vi "Start Tasks.vi"(8 "error in (no error)":errorcluster, 11 "Series Actor in":refnum<class "Series Actor.lvclass">) -> (0 "error out":errorcluster, 3 "Series Actor out":refnum<class "Series Actor.lvclass">)   [LabVIEW 2023, in "Series Actor.lvlib" / "Series Actor.lvclass"]
uses:
  Series Actor.lvclass
  C:/Program Files/National Instruments/LabVIEW 2023/vi.lib/ActorFramework/Actor/Actor.lvclass
  Task/Task Actor/Task Actor/Task Actor/Task Actor.lvclass
  Series Actor.lvclass/Series Actor.ctl
  Series Base/Series Base.lvclass/Series Base.ctl
  Task/Task Actor/Task Actor/Task Actor/Task Actor.lvclass/Task Actor.ctl
  <vilib>/ActorFramework/Message Enqueuer/Message Enqueuer.lvclass/Message Enqueuer.ctl
  <vilib>/ActorFramework/Message Enqueuer/Enqueue.vi
  Task/Task Actor/ITask Actor/ITask Actor Messages/Perform Action Msg/Perform Action Msg.lvclass
  C:/Program Files/National Instruments/LabVIEW 2023/vi.lib/ActorFramework/Message/Message.lvclass
  <vilib>/Utility/LVClass/Get LV Class Name.vi
  <resource>/AFDebug/Generate Trace for Message.vi
  <vilib>/ActorFramework/Message Priority Queue/Priority Enqueue.vi
  Series Base/Series Base.lvclass
  <vilib>/ActorFramework/Actor/Actor.lvclass
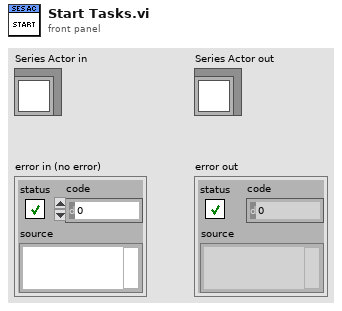
[diagram p1: front panel]
types:
  T1 = map{string, refnum<class "Message Enqueuer.lvclass">}
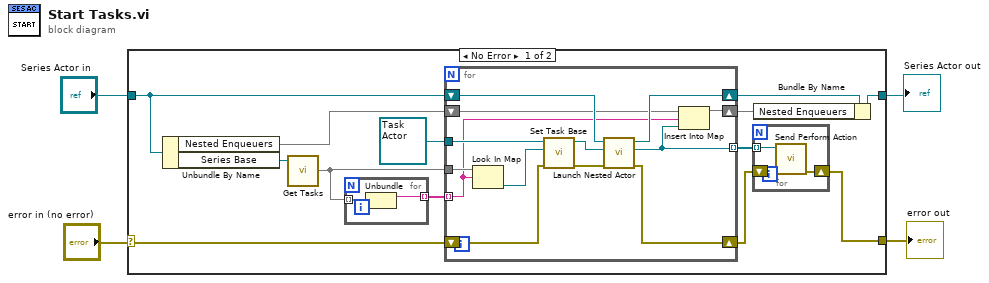
[diagram p0: block diagram]
diagram:
  n1 = case shown="No Error" "error in (no error)" {
    selector: "error in (no error)" -> [w5 w37]
    tunnel: "Series Actor in" -> [w14 w36]
    tunnel: [w10 w36] -> w3
    tunnel: [w6 w37] -> w2
    frame No Error {
      n2 = Unbundle By Name(w14) -> ("Nested Enqueuers"=w11:T1, "Series Base"=w17:refnum<class "Series Base.lvclass">)
      n3 = call "Get Tasks.vi"("HAL GOOP4:Series Base in"=w17) -> ("Tasks"=w16:map{string, refnum<class "Task Base.lvclass">})  [unwired: 8 in, 2 out]
      n4 = for {
        tunnel: w16 -> [w35] mode=indexing
        tunnel: [w34] -> w15 mode=indexing
        n5 = Unbundle(w35) -> (w34:string)  [unwired: 1 out]
      }
      n6 = for {
        tunnel: w16 -> [w33]
        tunnel: w15 -> [w23] mode=indexing
        shift-right: [w25] -> w12
        shift-left: w14 -> [w32]
        tunnel: refnum<class "Task Actor.lvclass"> refnum ("Task Actor.lvlib:Task Actor.lvclass") -> [w31]
        shift-right: [w26] -> w7
        shift-left: w5 -> [w28]
        shift-right: [w22] -> w9
        shift-left: w11 -> [w24]
        tunnel: [w21] -> w8 mode=indexing
        n7 = Look In Map(map=w33, key=w23) -> (value=w29:refnum<class "Task Base.lvclass">)  [unwired: 1 in, 1 out]
        n8 = call "Set Task Base.vi"("error in (no error)"=w28, "HAL GOOP4.lvlib:Task Base.lvclass"=w29, "Task Actor in"=w31) -> ("error out"=w27:errorcluster, "Task Actor out"=w30:refnum<class "Task Actor.lvclass">)  [unwired: 7 in]
        n9 = call <vilib>:"Launch Nested Actor.vi"("error in (no error)"=w27, "Nested Actor"=w30, "Caller Actor in"=w32) -> ("error out"=w26:errorcluster, "Nested Actor's Enqueuer"=w21:refnum<class "Message Enqueuer.lvclass">, "Caller Actor out"=w25:refnum<class "Series Actor.lvclass">)  [unwired: 6 in]
        n10 = Insert Into Map(map in=w24, key=w23, value=w21) -> (map out=w22:T1)  [unwired: 2 out]
      }
      n11 = for {
        tunnel: w8 -> [w20] mode=indexing
        shift-right: [w18] -> w6
        shift-left: w7 -> [w19]
        n12 = call "Send Perform Action.vi"("error in (no error)"=w19, "Message Enqueuer"=w20) -> ("error out"=w18:errorcluster)  [unwired: 8 in, 1 out]
      }
      n13 = Bundle By Name(cluster=w12, "Nested Enqueuers"=w9) -> (w10:refnum<class "Series Actor.lvclass">)
    }
    frame Error {
    }
  }
  "error out" <- w2
  "Series Actor out" <- w3
